vi "ReinstateNaNs.vi"(10 "DataIn":T1, 11 "TargetLength":i32) -> (3 "PlotData":dbl[][](array[numeric]))   [LabVIEW 2016]
doc: "Restores NaN values where sanitisation has trimmed them out, in order to preserve alignment with pressure data"
panel:
  # "Vmag"
  # "U"
  # "V"
  # "W"
  # "Cone"
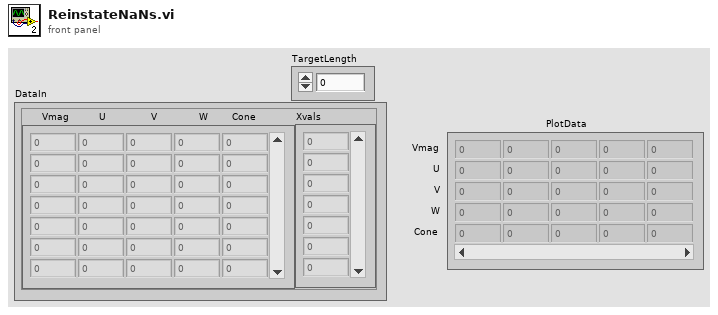
[diagram p1: front panel]
types:
  T1 = cluster{"   Vmag          U               V              W        Cone":dbl[][], "Xvals":i32[]}
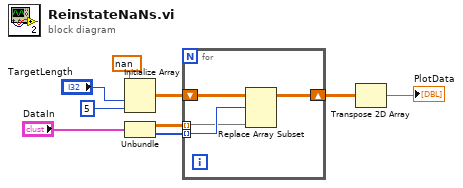
[diagram p0: block diagram]
diagram:
  n1 = Initialize Array(nan ("element"), "TargetLength", 5 ("dimension size")) -> (w2:dbl[][])
  n2 = Unbundle("DataIn") -> ("Vmag          U               V              W        Cone"=w8:dbl[][], "Xvals"=w7:i32[])
  n3 = for {
    tunnel: w8 -> [w12] mode=indexing
    tunnel: w7 -> [w13] mode=indexing
    shift-right: [w11] -> w3
    shift-left: w2 -> [w10]
    n4 = Replace Array Subset(array=w10, new element=w12, index (row)=w13) -> (w11:dbl[][])  [unwired: 1 in]
  }
  n5 = Transpose 2D Array(2D array=w3) -> (transposed array=→"PlotData":dbl[][])
